vi "Create Default Config settings.vi"(8 "error in":errorcluster, 11 "Config File Ref":T4) -> (0 "error out":errorcluster, 2 "Configuration Data":T1={"Plugin Configuration Information"={"Plugin Locaiton on Disk"=path ""}, "UI Configuration Information"={"Space Between Buttons"=3, "Number of Buttons to Show"=6, "Header Image"=path "Images/Blue Background.bmp", "Footer Image"=path "Images/Blue Background.bmp"}}, 3 "refnum out":T4)   [LabVIEW 2011]
uses:
  <vilib>/Utility/config.llb/Config Data RefNum.ctl
  Main Type Definitions/Framework Configuration Data.ctl
  Plugin Handler/Plugin Strict Type Definitions/Plugin Configuration Information.ctl
  User Interface/UI Control Definitions/UI Configuration Information.ctl
  <vilib>/Utility/config.llb/Read Key (Path).vi
  <vilib>/Utility/config.llb/Write Key (Path).vi
  <vilib>/Utility/config.llb/Read Key (I32).vi
  <vilib>/Utility/config.llb/Write Key (I32).vi
  <vilib>/Utility/config.llb/NI_LVConfig.lvlib
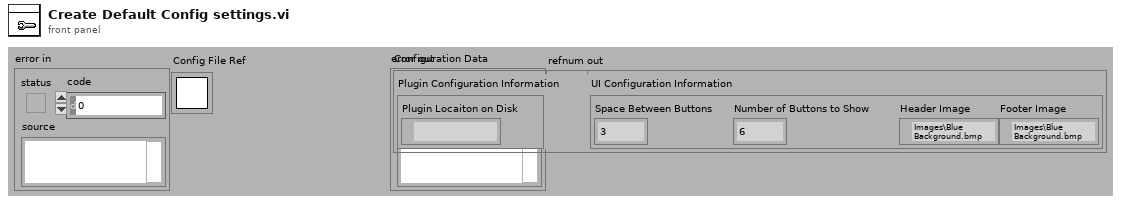
[diagram p1: front panel]
types:
  T1 = typedef "Framework Configuration Data.ctl" = cluster{"Plugin Configuration Information":T2, "UI Configuration Information":T3}
  T2 = typedef "Plugin Configuration Information.ctl" = cluster{"Plugin Locaiton on Disk":path}
  T3 = typedef "UI Configuration Information.ctl" = cluster{"Space Between Buttons":i32, "Number of Buttons to Show":i32, "Header Image":path, "Footer Image":path}
  T4 = typedef "NI_LVConfig.lvlib/Config Data RefNum.ctl" = refnum<k1>
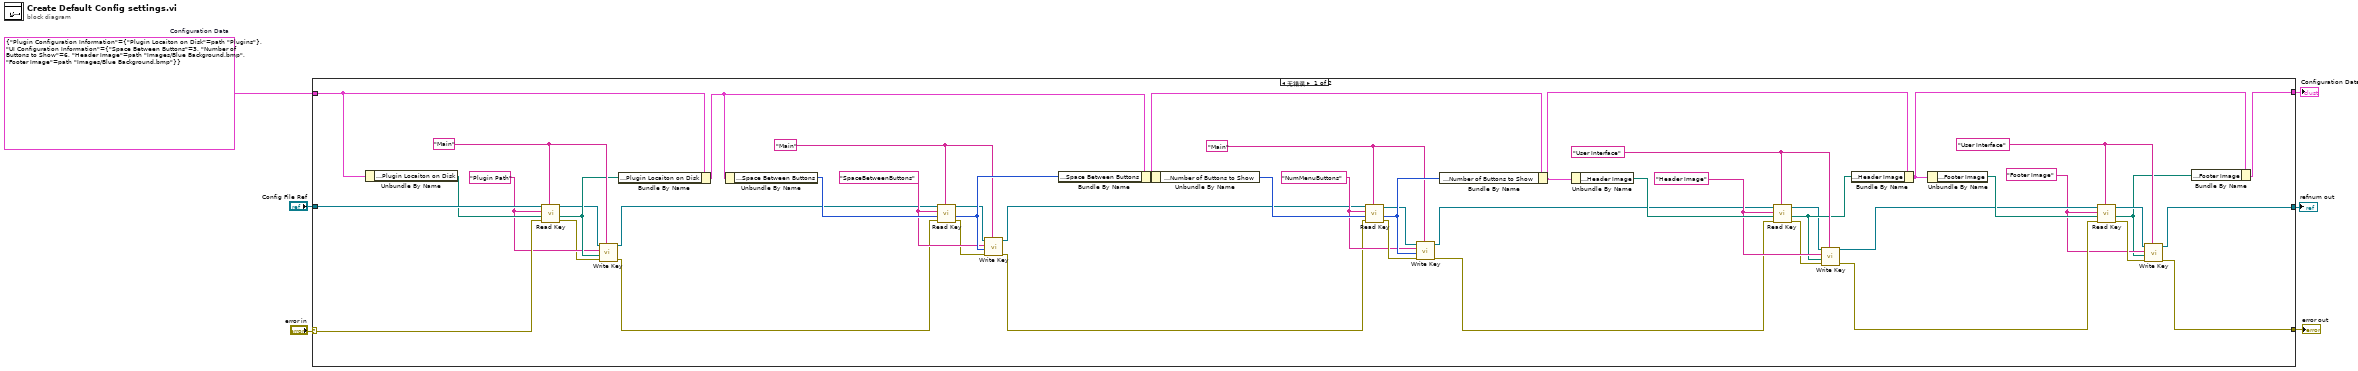
[diagram p0: block diagram]
diagram:
  w2 = T1 {"Plugin Configuration Information"={"Plugin Locaiton on Disk"=path "Plugins"}, "UI Configuration Information"={"Space Between Buttons"=3, "Number of Buttons to Show"=6, "Header Image"=path "Images/Blue Background.bmp", "Footer Image"=path "Images/Blue Background.bmp"}}  # Configuration Data
  n1 = case shown="无错误" "error in" {
    selector: "error in" -> [w51 w57]
    tunnel: [w33 w57] -> w4
    tunnel: "Config File Ref" -> [w54 w56]
    tunnel: [w31 w56] -> w3
    tunnel: w2 -> [w52 w55]
    tunnel: [w42 w55] -> w1
    frame No Error {
      w24 = "Main" ("section")
      w18 = "Main" ("section")
      w23 = "NumMenuButtons"
      w19 = "SpaceBetweenButtons"
      w13 = "Main" ("section")
      w11 = "Plugin Path" ("key")
      w29 = "Footer Image" ("key")
      w30 = "User Interface" ("section")
      w41 = "Header Image" ("key")
      w40 = "User Interface" ("section")
      n2 = Unbundle By Name(w52) -> ("Plugin Configuration Information.Plugin Locaiton on Disk"=w53:path)
      n3 = call-poly <vilib>:"Read Key.vi"("section"=w13, "error in (no error)"=w51, "default value"=w53, "key"=w11, "refnum"=w54) -> ("error out"=w10:errorcluster, "value"=w12:path, "refnum out"=w8:T4)  [unwired: 3 in, 1 out]
      n4 = call-poly <vilib>:"Write Key.vi"("section"=w13, "error in (no error)"=w10, "value"=w12, "key"=w11, "refnum"=w8) -> ("error out"=w9:errorcluster, "refnum out"=w7:T4)  [unwired: 4 in, 1 out]
      n5 = Bundle By Name(cluster=w52, "Plugin Configuration Information.Plugin Locaiton on Disk"=w12) -> (w49:T1)
      n6 = Unbundle By Name(w49) -> ("UI Configuration Information.Space Between Buttons"=w50:i32)
      n7 = call-poly <vilib>:"Read Key.vi"("section"=w18, "error in (no error)"=w9, "default value"=w50, "key"=w19, "refnum"=w7) -> ("error out"=w15:errorcluster, "value"=w20:i32, "refnum out"=w17:T4)  [unwired: 3 in, 1 out]
      n8 = call-poly <vilib>:"Write Key.vi"("section"=w18, "error in (no error)"=w15, "value"=w20, "key"=w19, "refnum"=w17) -> ("error out"=w14:errorcluster, "refnum out"=w16:T4)  [unwired: 4 in, 1 out]
      n9 = Bundle By Name(cluster=w49, "UI Configuration Information.Space Between Buttons"=w20) -> (w47:T1)
      n10 = Unbundle By Name(w47) -> ("UI Configuration Information.Number of Buttons to Show"=w48:i32)
      n11 = call-poly <vilib>:"Read Key.vi"("section"=w24, "error in (no error)"=w14, "default value"=w48, "key"=w23, "refnum"=w16) -> ("error out"=w27:errorcluster, "value"=w25:i32, "refnum out"=w22:T4)  [unwired: 3 in, 1 out]
      n12 = call-poly <vilib>:"Write Key.vi"("section"=w24, "error in (no error)"=w27, "value"=w25, "key"=w23, "refnum"=w22) -> ("error out"=w26:errorcluster, "refnum out"=w21:T4)  [unwired: 4 in, 1 out]
      n13 = Bundle By Name(cluster=w47, "UI Configuration Information.Number of Buttons to Show"=w25) -> (w45:T1)
      n14 = Unbundle By Name(w45) -> ("UI Configuration Information.Header Image"=w46:path)
      n15 = call-poly <vilib>:"Read Key.vi"("section"=w40, "error in (no error)"=w26, "default value"=w46, "key"=w41, "refnum"=w21) -> ("error out"=w36:errorcluster, "value"=w39:path, "refnum out"=w38:T4)  [unwired: 3 in, 1 out]
      n16 = call-poly <vilib>:"Write Key.vi"("section"=w40, "error in (no error)"=w36, "value"=w39, "key"=w41, "refnum"=w38) -> ("error out"=w35:errorcluster, "refnum out"=w37:T4)  [unwired: 4 in, 1 out]
      n17 = Bundle By Name(cluster=w45, "UI Configuration Information.Header Image"=w39) -> (w43:T1)
      n18 = Unbundle By Name(w43) -> ("UI Configuration Information.Footer Image"=w44:path)
      n19 = call-poly <vilib>:"Read Key.vi"("section"=w30, "error in (no error)"=w35, "default value"=w44, "key"=w29, "refnum"=w37) -> ("error out"=w34:errorcluster, "value"=w28:path, "refnum out"=w32:T4)  [unwired: 3 in, 1 out]
      n20 = call-poly <vilib>:"Write Key.vi"("section"=w30, "error in (no error)"=w34, "value"=w28, "key"=w29, "refnum"=w32) -> ("error out"=w33:errorcluster, "refnum out"=w31:T4)  [unwired: 4 in, 1 out]
      n21 = Bundle By Name(cluster=w43, "UI Configuration Information.Footer Image"=w28) -> (w42:T1)
    }
    frame Error {
    }
  }
  "error out" <- w4
  "refnum out" <- w3
  "Configuration Data" <- w1
